vi "Project 6 Front ENd.vi"() -> ()   [LabVIEW 2019]
panel:
  in  "Signals":dynamicdata(graph)
  in  "OK Button":bool
  in  "stop":bool
  out "Velocity v(t)":cluster{"X":dbl[], "Y":dbl[]}[](graph) caption="XY Graph"
  out "Pos x(t)":cluster{"X":dbl[], "Y":dbl[]}[](graph) caption="XY Graph"
  out "Exp fit":cluster{"X":dbl[], "Y":dbl[]}[](graph) caption="XY Graph"
  out "Raw Data\nCentered\nfrom mean":cluster{"X":dbl[], "Y":dbl[]}[](graph) caption="XY Graph"
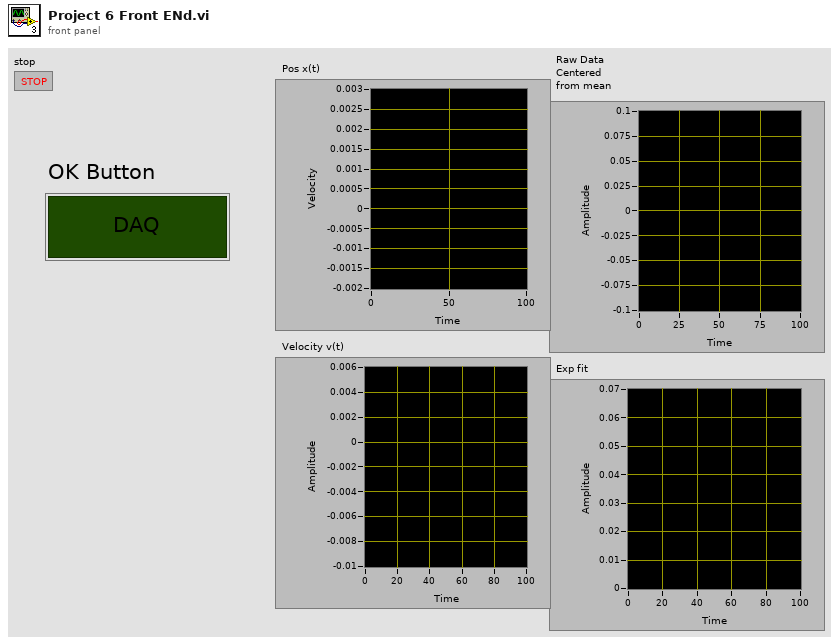
[diagram p1: front panel]
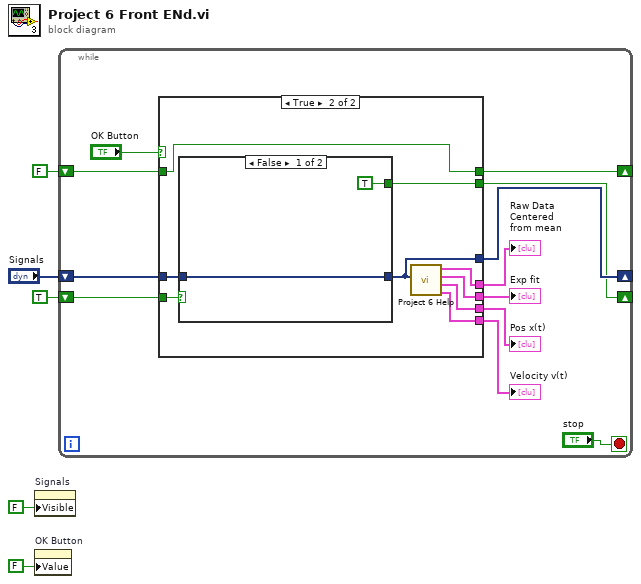
[diagram p0: block diagram]
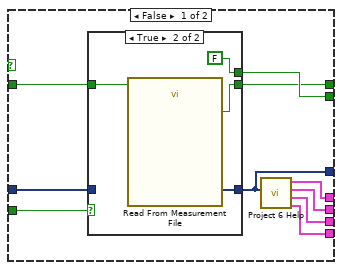
[diagram p2: hidden frame]
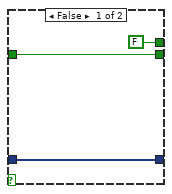
[diagram p3: hidden frame]
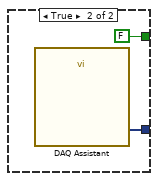
[diagram p4: hidden frame]
diagram:
  n1 = property on="Signals" class="WFGraph (strict)"("Visible"=FALSE) -> ()  [unwired: 2 in, 2 out]
  n2 = property on="OK Button" class="Bool (strict)"("Value"=FALSE ("OK Button")) -> ()  [unwired: 2 in, 2 out]
  n3 = while {
    shift-right: [w10] -> _
    shift-left: FALSE -> [w11]
    shift-right: [w7] -> _
    shift-left: TRUE -> [w9]
    shift-right: [w8] -> _
    shift-left: "Signals" -> [w6]
    stop <- "stop" stop-if-true
    n4 = case shown="True" "OK Button" {
      tunnel: [w27 w43] -> w17
      tunnel: [w26 w42] -> w16
      tunnel: [w25 w41] -> w15
      tunnel: [w24 w40] -> w14
      tunnel: w11 -> [w18 w35]
      tunnel: [w19 w35] -> w10
      tunnel: w9 -> [w23 w38]
      tunnel: [w22 w39] -> w8
      tunnel: [w21 w37] -> w7
      tunnel: w6 -> [w20 w36]
      frame False {
        n5 = case shown="True" w23 {
          tunnel: [w30 w34] -> w22
          tunnel: [FALSE FALSE] -> w21
          tunnel: w20 -> [w30 _]
          tunnel: w18 -> [w28 w32]
          tunnel: [w28 w31] -> w19
          frame False {
          }
          frame True {
            n6 = call "Read From Measurement File"("Reset"=w32) -> ("Signals"=w34:dynamicdata, "EOF?"=w31:bool)  [unwired: 5 in, 4 out]
          }
        }
        n7 = call "Project 6 Help.vi"("Signals"=w22) -> ("Velocity v(t)"=w24:cluster{"X":dbl[], "Y":dbl[]}[], "Pos x(t)"=w25:cluster{"X":dbl[], "Y":dbl[]}[], "Exp fit"=w26:cluster{"X":dbl[], "Y":dbl[]}[], "Raw Data\nCentered\nfrom mean"=w27:cluster{"X":dbl[], "Y":dbl[]}[])  [unwired: 6 in, 1 out]
      }
      frame True {
        n8 = case shown="False" w38 {
          tunnel: [w44 w47] -> w39
          tunnel: [TRUE FALSE] -> w37
          tunnel: w36 -> [w44 _]
          frame False {
          }
          frame True {
            n9 = call "DAQ Assistant"() -> ("data"=w47:dynamicdata)  [unwired: 16 in, 3 out]
          }
        }
        n10 = call "Project 6 Help.vi"("Signals"=w39) -> ("Velocity v(t)"=w40:cluster{"X":dbl[], "Y":dbl[]}[], "Pos x(t)"=w41:cluster{"X":dbl[], "Y":dbl[]}[], "Exp fit"=w42:cluster{"X":dbl[], "Y":dbl[]}[], "Raw Data\nCentered\nfrom mean"=w43:cluster{"X":dbl[], "Y":dbl[]}[])  [unwired: 6 in, 1 out]
      }
    }
    "Raw Data\nCentered\nfrom mean" <- w17
    "Exp fit" <- w16
    "Pos x(t)" <- w15
    "Velocity v(t)" <- w14
  }
